vi "configuration.vi"(4 "custom_path":path, 6 "force_read?":bool, 7 "command":T1=enum."read_config", 8 "error in (no error)":errorcluster, 10 "project_file":path, 11 "config in":T2) -> (0 "error out":errorcluster, 3 "config out":T2)   [LabVIEW 2015, in "lv-build.lvlib"]
uses:
  lv-build.lvlib
  _controls/configuration.ctl
  _controls/configuration_command.ctl
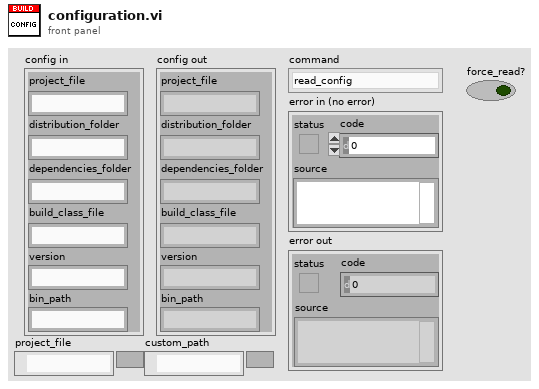
[diagram p1: front panel]
types:
  T1 = typedef "lv-build.lvlib/configuration_command.ctl" = enum16{"<config_command>", "read_config", "write_config", "<null>"}
  T2 = typedef "lv-build.lvlib/configuration.ctl" = cluster{"project_file":string, "distribution_folder":string, "dependencies_folder":string, "build_class_file":string, "version":string, "bin_path":string}
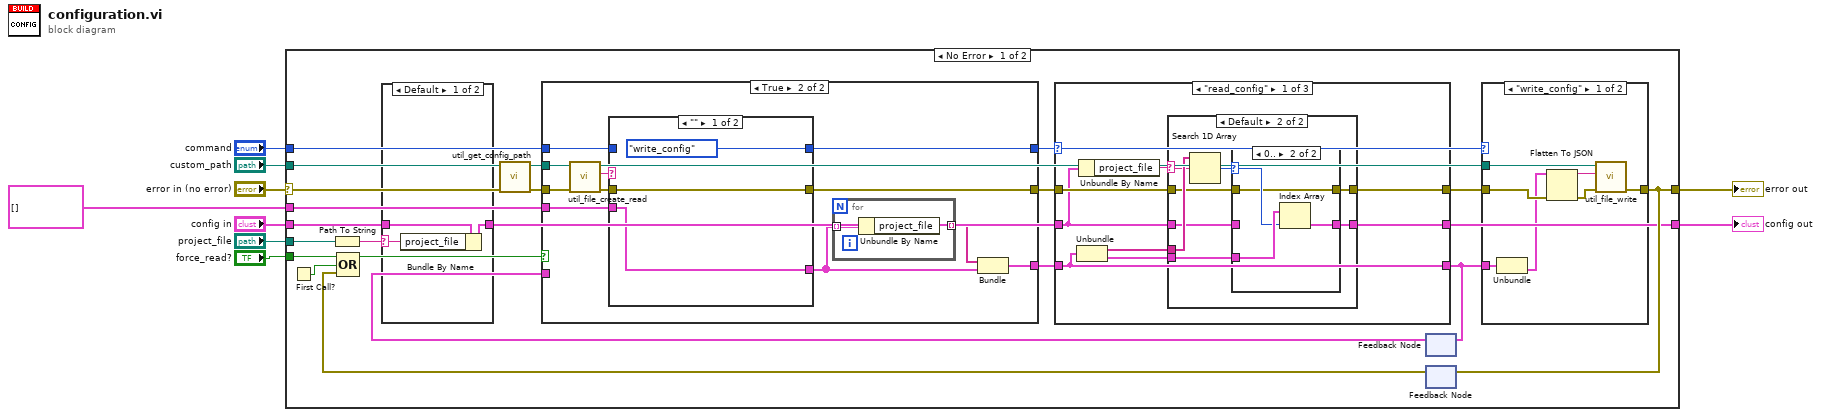
[diagram p0: block diagram]
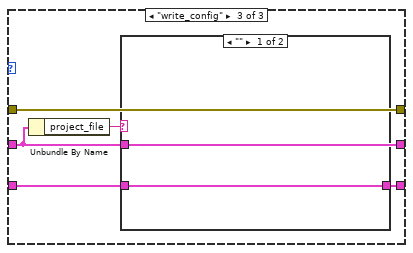
[diagram p6: hidden frame]
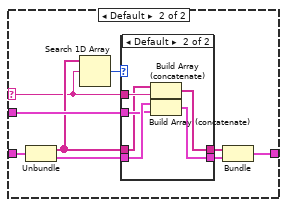
[diagram p7: hidden frame]
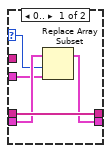
[diagram p8: hidden frame]
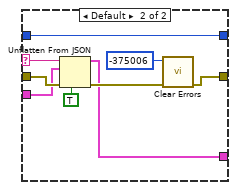
[diagram p10: hidden frame]
diagram:
  n1 = case shown="No Error" "error in (no error)" {
    selector: "error in (no error)" -> [w23 w125]
    tunnel: "command" -> [w25 _]
    tunnel: [w31 w125] -> w6
    tunnel: "config in" -> [w12 _]
    tunnel: "force_read?" -> [w28 _]
    tunnel: T2[] [] -> [w26 _]
    tunnel: [w17 _] -> w3
    tunnel: "project_file" -> [w14 _]
    tunnel: "custom_path" -> [w10 _]
    frame No Error {
      n2 = First Call?() -> (First Call?: T/F=w29:bool)
      n3 = Path To String(path=w14) -> (string=w13:string)
      n4 = case shown="Default" w13 {
        selector: w13 -> [w33 _]
        tunnel: w12 -> [w34 w35]
        tunnel: [w32 w35] -> w11
        frame Default {
          n5 = Bundle By Name(cluster=w34, "project_file"=w33) -> (w32:T2)
        }
        frame "" {
        }
      }
      n6 = call "util_get_config_path.vi"("error in (no error)"=w23, "custom_path"=w10) -> ("error out"=w22:errorcluster, "lv_build_config_path"=w24:path)  [unwired: 8 in]
      n7 = feedback #1() -> (w21:cluster{string[], T2[]})  [unwired: 1 in]
      n8 = feedback #2() -> (w30:errorcluster)  [unwired: 1 in]
      n9 = Compound Arithmetic op=OR(w28, w29, w30) -> (w27:bool)
      n10 = case shown="True" w27 {
        tunnel: w21 -> [w89 _]
        tunnel: w22 -> [w91 w100]
        tunnel: w24 -> [_ w101]
        tunnel: [w91 w98] -> w16
        tunnel: w26 -> [_ w102]
        tunnel: w25 -> [w90 w97]
        tunnel: [w90 w96] -> w18
        tunnel: [w89 w93] -> w19
        frame False {
        }
        frame True {
          n11 = call "util_file_create_read.vi"("error in (no error)"=w100, "config_path"=w101) -> ("error out"=w99:errorcluster, "string"=w95:string)  [unwired: 8 in]
          n12 = case shown="\"\"" w95 {
            selector: w95 -> [_ w114]
            tunnel: w102 -> [w106 w115]
            tunnel: [w106 w108] -> w94
            tunnel: w99 -> [w107 w116]
            tunnel: [w107 w109] -> w98
            tunnel: w97 -> [_ w113]
            tunnel: [configuration_command."write_config" ("command") w113] -> w96
            frame "" {
            }
            frame Default {
              n13 = Unflatten From JSON(JSON string=w114, type and defaults=w115, default null elements? (F)=TRUE, error in (no error)=w116) -> (value=w108:T2[], error out=w111:errorcluster)  [unwired: 3 in]
              n14 = call <vilib>:"Clear Errors.vi"("error in (no error)"=w111, "specific error code to clear (0: all)"=-375006) -> ("error out"=w109:errorcluster)  [unwired: 4 in, 1 out]
            }
          }
          n15 = for {
            tunnel: w94 -> [w104] mode=indexing
            tunnel: [w103] -> w92 mode=indexing
            n16 = Unbundle By Name(w104) -> ("project_file"=w103:string)
          }
          n17 = Bundle(w92, w94) -> (w93:cluster{string[], T2[]})  [unwired: 1 in]
        }
      }
      n18 = case shown="\"read_config\"" w18 {
        tunnel: w11 -> [w36 w62 w64]
        tunnel: [w43 w61 w67] -> w20
        tunnel: w19 -> [w43 w61 w65]
        tunnel: [w39 w62 w64] -> w17
        tunnel: w16 -> [w38 w60 w63]
        tunnel: [w37 w60 w63] -> w15
        frame "read_config" {
          n19 = Unbundle(w43) -> (w42:string[], w41:T2[])
          n20 = Unbundle By Name(w36) -> ("project_file"=w40:string)
          n21 = case shown="Default" w40 {
            selector: w40 -> [_ w50]
            tunnel: w42 -> [_ w53]
            tunnel: w41 -> [_ w52]
            tunnel: [w44 w49] -> w39
            tunnel: w38 -> [w45 w48]
            tunnel: [w45 w47] -> w37
            tunnel: w36 -> [w44 w46]
            frame "" {
            }
            frame Default {
              n22 = Search 1D Array(1D array=w53, element=w50) -> (index of element=w51:i32)  [unwired: 1 in]
              n23 = case shown="0.." w51 {
                selector: w51 -> [_ w58]
                tunnel: w52 -> [_ w59]
                tunnel: [w54 w57] -> w49
                tunnel: w48 -> [w55 w56]
                tunnel: [w55 w56] -> w47
                tunnel: w46 -> [w54 _]
                frame Default {
                }
                frame 0.. {
                  n24 = Index Array(array=w59, index=w58) -> (element=w57:T2)
                }
              }
            }
          }
        }
        frame Default {
        }
        frame "write_config" {
          n25 = Unbundle By Name(w64) -> ("project_file"=w66:string)
          n26 = case shown="\"\"" w66 {
            selector: w66 -> [_ w69]
            tunnel: [w68 w75] -> w67
            tunnel: w64 -> [_ w73]
            tunnel: w65 -> [w68 w71]
            frame "" {
            }
            frame Default {
              n27 = Unbundle(w71) -> (w70:string[], w72:T2[])
              n28 = Search 1D Array(1D array=w70, element=w69) -> (index of element=w77:i32)  [unwired: 1 in]
              n29 = case shown="Default" w77 {
                selector: w77 -> [w78 _]
                tunnel: w72 -> [w81 w87]
                tunnel: [w80 w85] -> w76
                tunnel: w70 -> [w82 w83]
                tunnel: [w82 w84] -> w74
                tunnel: w73 -> [w79 w86]
                tunnel: w69 -> [_ w88]
                frame 0.. {
                  n30 = Replace Array Subset(array=w81, new element=w79, index=w78) -> (w80:T2[])
                }
                frame Default {
                  n31 = Build Array (concatenate)(w83, w88) -> (w84:string[])
                  n32 = Build Array (concatenate)(w87, w86) -> (w85:T2[])
                }
              }
              n33 = Bundle(w74, w76) -> (w75:cluster{string[], T2[]})  [unwired: 1 in]
            }
          }
        }
      }
      n34 = feedback-in #1(w20) -> ()
      n35 = case shown="\"write_config\"" w18 {
        tunnel: w20 -> [w118 _]
        tunnel: w15 -> [w121 w124]
        tunnel: [w119 w124] -> w31
        tunnel: w24 -> [w120 _]
        frame "write_config" {
          n36 = Unbundle(w118) -> (w117:T2[])  [unwired: 1 out]
          n37 = Flatten To JSON(anything=w117, error in (no error)=w121) -> (JSON string=w123:string, 11:w122:errorcluster)  [unwired: 1 in]
          n38 = call "util_file_write.vi"("error in (no error)"=w122, "string"=w123, "config_path"=w120) -> ("error out"=w119:errorcluster)  [unwired: 8 in]
        }
        frame Default {
        }
      }
      n39 = feedback-in #2(w31) -> ()
    }
    frame Error {
      # "If an error is wired in, be sure to skip over functionality to preserve the original error"
    }
  }
  "config out" <- w3
  "error out" <- w6
